vi "set_config_cluster.vi"(8 "error in (no error)":errorcluster, 10 "config cluster variant":variant, 11 "ClockDL100201DAQmx in":refnum<class "ClockDL100201DAQmx.lvclass">) -> (0 "error out":errorcluster, 3 "ClockDL100201DAQmx out":refnum<class "ClockDL100201DAQmx.lvclass">)   [LabVIEW 2010, in "ClockDL100201DAQmx.lvclass"]
uses:
  ClockDL100201DAQmx.lvclass
  ClockDL100201DAQmx.lvclass/ClockDL100201DAQmx.ctl
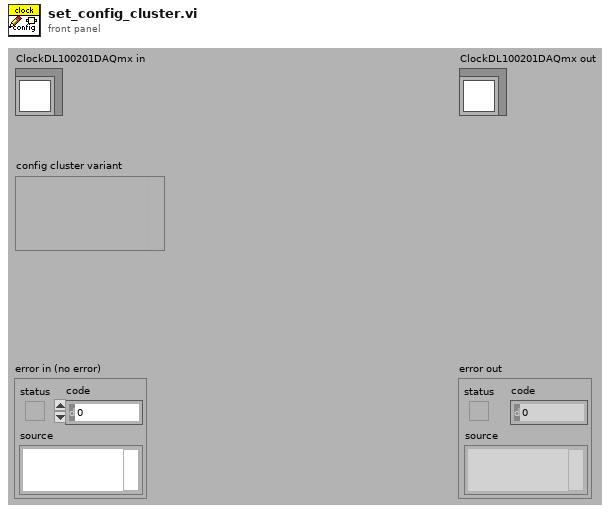
[diagram p1: front panel]
types:
  T1 = typedef "ClockDL100201DAQmx.lvclass/config_data_cluster.ctl" = cluster{"source":string, "destination":string, "counter":string}
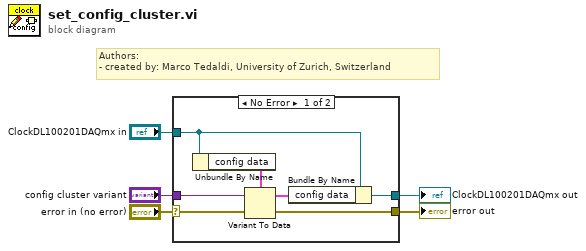
[diagram p0: block diagram]
diagram:
  # "Authors: \n- created by: Marco Tedaldi, University of Zurich, Switzerland"
  n1 = case shown="No Error" "error in (no error)" {
    selector: "error in (no error)" -> [w12 w14]
    tunnel: [w11 w14] -> w4
    tunnel: "ClockDL100201DAQmx in" -> [w8 w13]
    tunnel: "config cluster variant" -> [w10 _]
    tunnel: [w6 w13] -> w1
    frame No Error {
      n2 = Unbundle By Name(w8) -> ("config data"=w7:T1)
      n3 = Variant To Data(error in=w12, Variant=w10, type=w7) -> (error out=w11:errorcluster, data=w9:T1)
      n4 = Bundle By Name(cluster=w8, "config data"=w9) -> (w6:refnum<class "ClockDL100201DAQmx.lvclass">)
    }
    frame Error {
    }
  }
  "error out" <- w4
  "ClockDL100201DAQmx out" <- w1
